vi "save_config_file.vi"(8 "error in (no error)":errorcluster, 9 "config cluster variant":variant, 11 "DL090216RangeOffsetImageProcessor in":refnum<class "ImageProcessorDL090216RangeOffset.lvclass">) -> (0 "error out":errorcluster, 3 "DL090216RangeOffsetImageProcessor out":refnum<class "ImageProcessorDL090216RangeOffset.lvclass">)   [LabVIEW 2010]
uses:
  ImageProcessorDL090216RangeOffset.lvclass
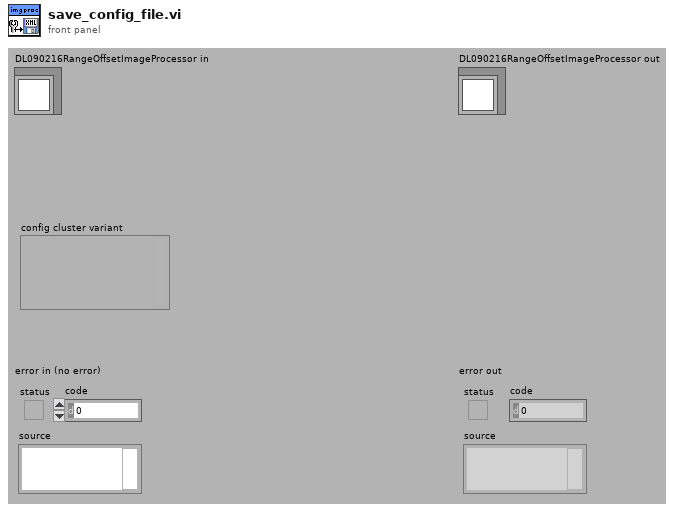
[diagram p1: front panel]
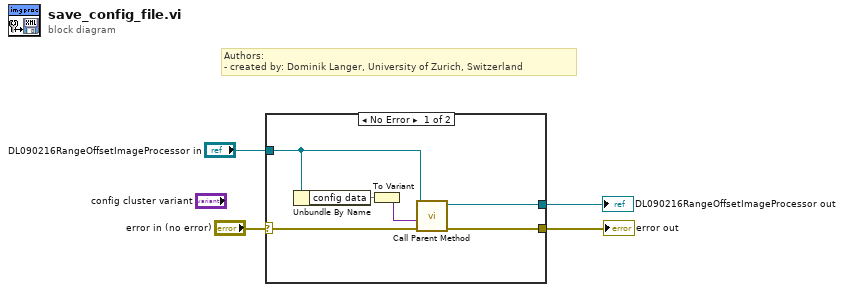
[diagram p0: block diagram]
diagram:
  # "Authors: \n- created by: Dominik Langer, University of Zurich, Switzerland"
  n1 = case shown="No Error" "error in (no error)" {
    selector: "error in (no error)" -> [w5 w11]
    tunnel: [w10 w11] -> w4
    tunnel: [w9 w12] -> w3
    tunnel: "DL090216RangeOffsetImageProcessor in" -> [w8 w12]
    frame No Error {
      n2 = Unbundle By Name(w8) -> ("config data"=w7)
      n3 = To Variant(anything=w7) -> (Variant=w6:variant)
      n4 = call-parent "Call Parent Method"("error in (no error)"=w5, "config cluster variant"=w6, "GenericPlugin in"=w8) -> ("error out"=w10:errorcluster, "GenericPlugin out"=w9:refnum<class "ImageProcessorDL090216RangeOffset.lvclass">)  [unwired: 1 in, 6 out]
    }
    frame Error {
    }
  }
  "error out" <- w4
  "DL090216RangeOffsetImageProcessor out" <- w3
